vi "getPieceAngle.vi"(1 "Center Num":dbl[](array[numeric]), 2 "Center Piece":dbl[](array[numeric])) -> (0 "Angle":dbl)   [LabVIEW 2016]
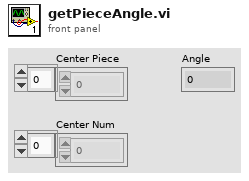
[diagram p1: front panel]
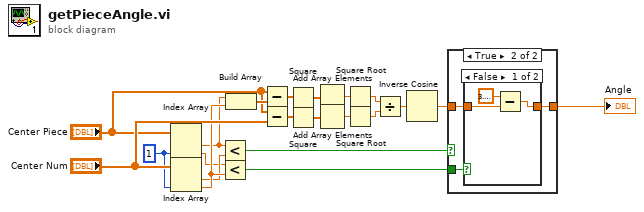
[diagram p0: block diagram]
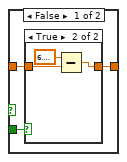
[diagram p2: hidden frame]
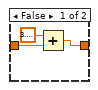
[diagram p3: hidden frame]
diagram:
  w1 = 1 ("index")
  n1 = Index Array(array="Center Piece", index #2=w1) -> (element #1=w4:dbl, element #2=w2:dbl)  [unwired: 1 in]
  n2 = Index Array(array="Center Num", index #2=w1) -> (element #1=w3:dbl, element #2=w5:dbl)  [unwired: 1 in]
  n3 = Less?(x=w4, y=w3) -> (x < y?=w6:bool)
  n4 = Less?(x=w2, y=w5) -> (x < y?=w7:bool)
  n5 = Build Array(w4, w5) -> (w15:dbl[])
  n6 = Subtract(x="Center Piece", y=w15) -> (x-y=w13:dbl[])
  n7 = Subtract(x="Center Piece", y="Center Num") -> (x-y=w8:dbl[])
  n8 = Square(x=w13) -> (x^2=w12:dbl[])
  n9 = Square(x=w8) -> (x^2=w9:dbl[])
  n10 = Add Array Elements(numeric array=w12) -> (sum=w11:dbl)
  n11 = Add Array Elements(numeric array=w9) -> (sum=w10:dbl)
  n12 = Square Root(x=w11) -> (sqrt(x)=w17:dbl)
  n13 = Square Root(x=w10) -> (sqrt(x)=w18:dbl)
  n14 = Divide(x=w17, y=w18) -> (x/y=w19:dbl)
  n15 = Inverse Cosine(1:w19) -> (0:w20:dbl)
  n16 = case shown="True" w6 {
    tunnel: w7 -> [w24 w33]
    tunnel: w20 -> [w23 w32]
    tunnel: [w22 w31] -> w21
    frame False {
      n17 = case shown="True" w24 {
        tunnel: w23 -> [w27 w30]
        tunnel: [w25 w28] -> w22
        frame False {
          n18 = Add(x=3.141592653589793, y=w27) -> (x+y=w25:dbl)
        }
        frame True {
          n19 = Subtract(x=6.283185307179586, y=w30) -> (x-y=w28:dbl)
        }
      }
    }
    frame True {
      n20 = case shown="False" w33 {
        tunnel: w32 -> [w36 w37]
        tunnel: [w34 w37] -> w31
        frame False {
          n21 = Subtract(x=3.141592653589793, y=w36) -> (x-y=w34:dbl)
        }
        frame True {
        }
      }
    }
  }
  "Angle" <- w21
